vi "_MDPtr Unpack Memory.vi"(10 "error in (no error)":errorcluster, 11 "HexStrPtr":T1) -> (1 "String Attribute":string, 2 "error out":errorcluster, 3 "string":string)   [LabVIEW 2017, in "MDPtr.lvlib"]
uses:
  MDPtr.lvlib
  MDPtr TypeDef/MDPtr.ctl
  MDPtr TypeDef/MDPtr DataFrame-Memory.ctl
  MDPtr TypeDef/MDPtr DataFrame-Common.ctl
  <vilib>/Utility/Data Type/Type Definitions/Data Type.ctl
  <vilib>/Utility/Data Type/NI_Data Type.lvlib
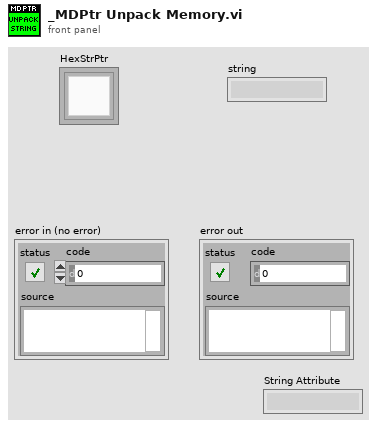
[diagram p1: front panel]
types:
  T1 = typedef "MDPtr.lvlib/MDPtr.ctl" = refnum<k1>
  T2 = typedef "MDPtr.lvlib/MDPtr DataFrame-Memory.ctl" = cluster{"Common":T3, "DVR":refnum<data-value>}
  T3 = typedef "MDPtr.lvlib/MDPtr DataFrame-Common.ctl" = cluster{"Data Type":T4, "Copy Count":i32, "String Attribute":string, "Cache Length":i32, "Data Length":i32}
  T4 = typedef "NI_Data Type.lvlib/Data Type.ctl" = enum8{"Invalid Type", "Void", "I8", "I16", "I32", "I64", "U8", "U16", "U32", "U64", "Single Float", "Double Float", "Extended Float", "Single Complex", "Double Complex", "Extended Complex", "Enum U8", "Enum U16", "Enum U32", "Enum U64", "Single Float With Unit", "Double Float With Unit", "Extended Float With Unit", "Single Complex with Unit", "Double Complex with Unit", "Extended Complex with Unit", "Boolean", "String", "Path", "Picture", "Tag", "Array", "Cluster", "Variant", "LV Variant", "Waveform", "Timestamp", "Digital Waveform", "Digital Data", "ExpressData", "Refnum", "External Data", "VI", "Poly VI", "LabVIEW Class Instance", "Fixed Point"}
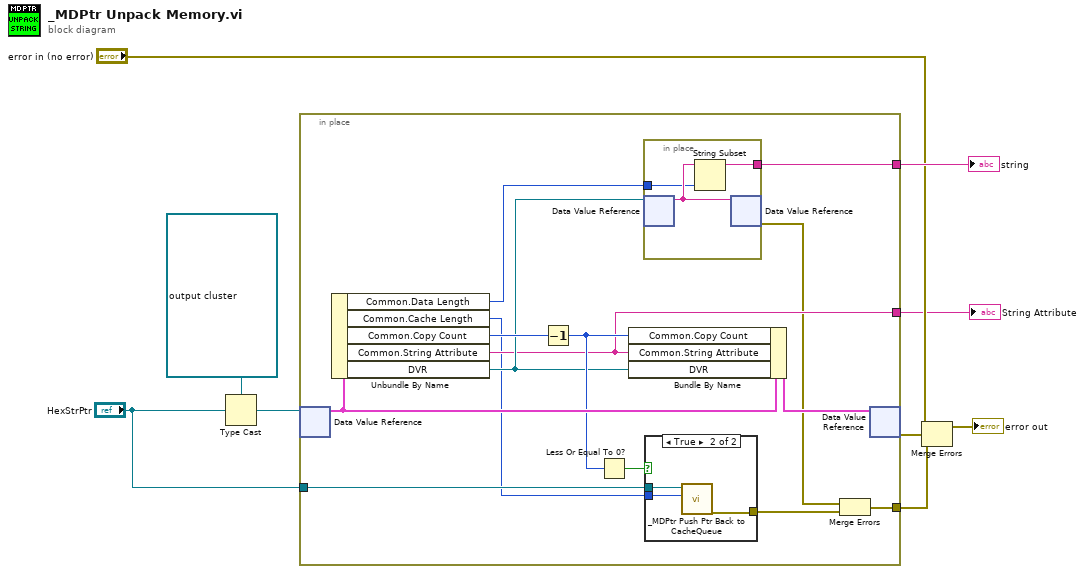
[diagram p0: block diagram]
diagram:
  n1 = Type Cast(type=refnum<data-value> refnum ("data value reference"), x="HexStrPtr") -> (*(type *) &x=w5:refnum<data-value>)
  n2 = in-place "In Place Element Structure" {
    in-place-border: [w20] -> w9
    in-place-border: [w17] -> w6
    in-place-border: "HexStrPtr" -> [w15]
    in-place-border: [w10] -> w1
    n3 = in-place-dvr #1(w5) -> (w23:T2)  [unwired: 1 out]
    n4 = Unbundle By Name(w23) -> ("Common.Data Length"=w14:i32, "Common.Cache Length"=w13:i32, "Common.Copy Count"=w21:i32, "Common.String Attribute"=w17:string, "DVR"=w18:refnum<data-value>)
    n5 = Decrement(x=w21) -> (x-1=w19:i32)
    n6 = Less Or Equal To 0?(x=w19) -> (x <= 0?=w16:bool)
    n7 = Bundle By Name(cluster=w23, "Common.Copy Count"=w19, "Common.String Attribute"=w17, "DVR"=w18) -> (w22:T2)
    n8 = in-place {
      in-place-border: [w28] -> w20
      in-place-border: w14 -> [w27]
      n9 = in-place-dvr #2(w18) -> (w29:string)  [unwired: 1 out]
      n10 = String Subset(string=w29, length (rest)=w27) -> (substring=w28:string)  [unwired: 1 in]
      n11 = in-place-dvr #2(w29) -> (w12:errorcluster)  [unwired: 1 out]
    }
    n12 = case shown="True" w16 {
      tunnel: [_ w26] -> w11
      tunnel: w15 -> [_ w24]
      tunnel: w13 -> [_ w25]
      frame False {
      }
      frame True {
        n13 = call "_MDPtr Push Ptr Back to CacheQueue.vi"("Cache Length"=w25, "MDPtr"=w24) -> ("error out"=w26:errorcluster)  [unwired: 9 in]
      }
    }
    n14 = Merge Errors(w12, w11) -> (w10:errorcluster)
    n15 = in-place-dvr #1(w22) -> (w2:errorcluster)  [unwired: 1 out]
  }
  "string" <- w9
  "String Attribute" <- w6
  n16 = Merge Errors("error in (no error)", w2, w1) -> (→"error out":errorcluster)
